vi "Get Category.vi"(8 "error in (no error)":errorcluster, 11 "Modbus Module editor node in":refnum<class "Modbus Module editor node.lvclass">) -> (0 "error out":errorcluster, 2 "Category":string, 3 "Modbus Module editor node out":refnum<class "Modbus Module editor node.lvclass">)   [LabVIEW 2015, in "Modbus Module editor node.lvclass"]
uses:
  Modbus Module editor node.lvclass
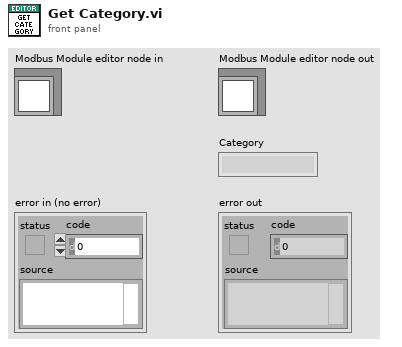
[diagram p1: front panel]
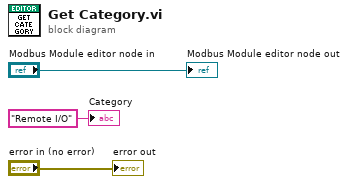
[diagram p0: block diagram]
diagram:
  "error out" <- "error in (no error)"
  "Modbus Module editor node out" <- "Modbus Module editor node in"
  "Category" <- "Remote I/O" ("Category")
